vi "await_console_close.vi"(8 "error in (no error)":errorcluster, 11 "console.provider in":refnum<class "console.provider.lvclass">) -> (0 "error out":errorcluster, 3 "console.provider out":refnum<class "console.provider.lvclass">)   [LabVIEW 2021, in "console.provider.lvclass"]
uses:
  console.provider.lvclass
  console.provider.lvclass/console.provider.ctl
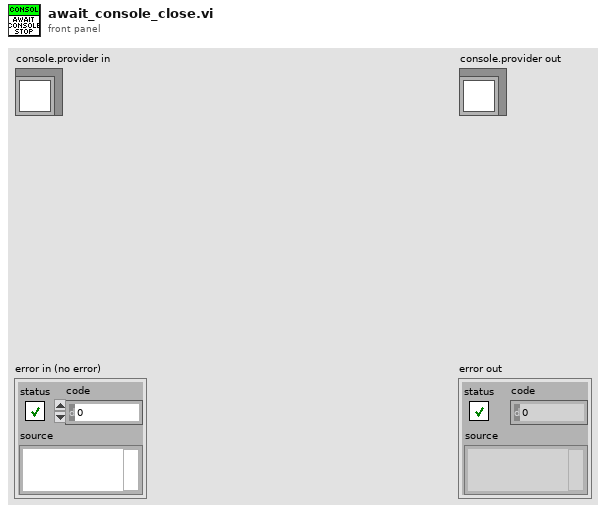
[diagram p1: front panel]
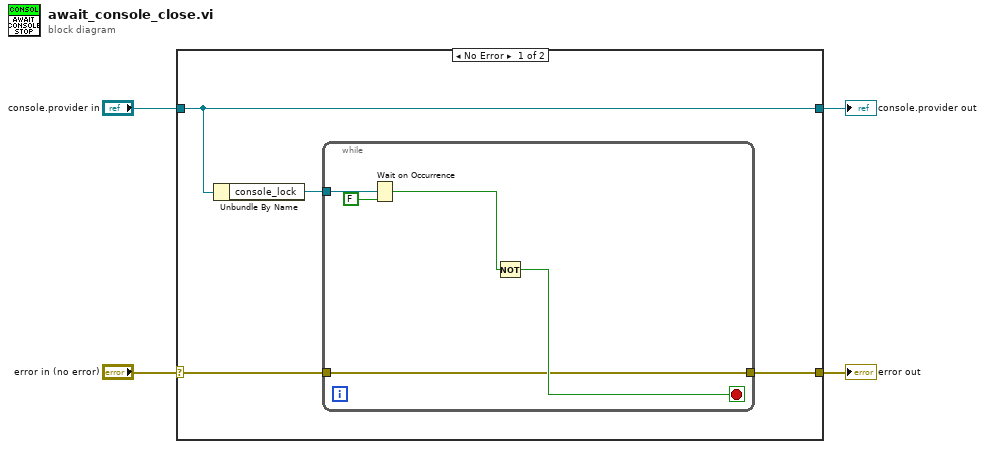
[diagram p0: block diagram]
diagram:
  n1 = case shown="No Error" "error in (no error)" {
    selector: "error in (no error)" -> [w6 w15]
    tunnel: [w5 w15] -> w1
    tunnel: [w8 w14] -> w3
    tunnel: "console.provider in" -> [w8 w14]
    frame No Error {
      n2 = Unbundle By Name(w8) -> ("console_lock"=w7:refnum<k4>)
      n3 = while {
        tunnel: w7 -> [w13]
        tunnel: w6 -> [w9]
        tunnel: [w9] -> w5
        stop <- w10 stop-if-true
        n4 = Wait on Occurrence(1:FALSE ("ignore previous (T)"), 2:w13) -> (0:w11:bool)  [unwired: 1 in]
        n5 = Not(x=w11) -> (.not. x?=w10:bool)
      }
    }
    frame Error {
    }
  }
  "error out" <- w1
  "console.provider out" <- w3
